vi "FTW-Endpoint-IncomingRequestProxy-Relay.vi"(0 "Incoming Request Event":refnum<user-event>, 5 "Frontend Endpoint":refnum<class "FTW-Endpoint-TCP.lvclass">, 7 "Multipart Message":string[](array[string]), 11 "error in":errorcluster) -> (4 "Incoming Request Event out":refnum<user-event>, 15 "error out":errorcluster)   [LabVIEW 2013, in "FTW-Endpoint-TCP.lvclass"]
uses:
  FTW-Endpoint-TCP.lvclass
  Message/Request/FTW-Message-IncomingRequest.lvclass
panel:
  # "Inputs"
  # "Outputs"
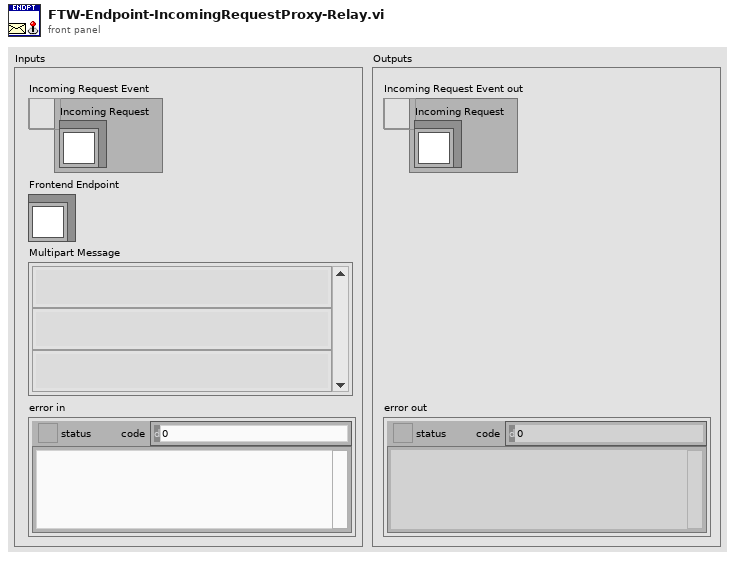
[diagram p1: front panel]
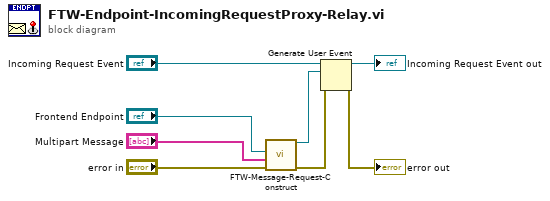
[diagram p0: block diagram]
diagram:
  n1 = call "FTW-Message-Request-Construct.vi"("error in"="error in", "Multipart Message"="Multipart Message", "Frontend Endpoint"="Frontend Endpoint") -> ("error out"=w2:errorcluster, "FTW Incoming Request"=w1:refnum<class "FTW-Message-IncomingRequest.lvclass">)  [unwired: 7 in]
  n2 = Generate User Event(user event="Incoming Request Event", event data cluster=w1, error in=w2) -> (user event out=→"Incoming Request Event out":refnum<user-event>, error out=→"error out":errorcluster)  [unwired: 1 in]
